vi "Update In World.vi"(11 "Chmmr in":refnum<class "Chmmr.lvclass">) -> (3 "Chmmr out":refnum<class "Chmmr.lvclass">)   [LabVIEW 2015, in "Chmmr.lvclass"]
uses:
  Chmmr.lvclass
  Element/Element.lvclass/Element.ctl
  Motion/Motion.lvclass/Motion.ctl
  Chmmr.lvclass/Chmmr.ctl
  <vilib>/Utility/High Resolution Relative Seconds.vi
  Ship/Ship.lvclass
  Math/Math.lvlib
  Motion/Motion.lvclass
  Element/Element.lvclass
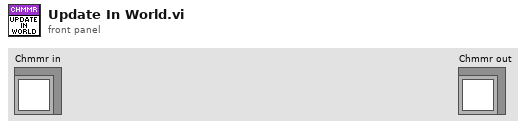
[diagram p1: front panel]
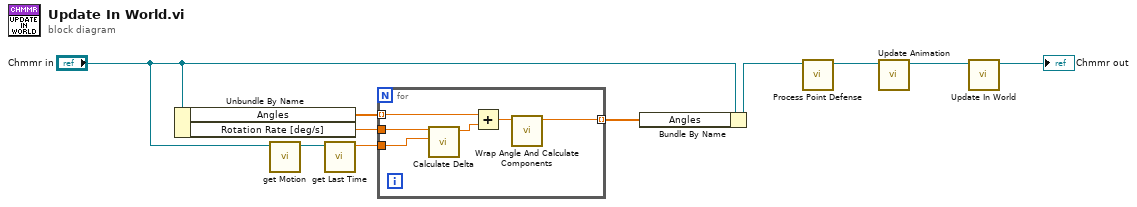
[diagram p0: block diagram]
diagram:
  n1 = Unbundle By Name("Chmmr in") -> ("Angles"=w10:sgl[], "Rotation Rate [deg/s]"=w8:sgl)
  n2 = call "get Motion.vi"("Movable in"="Chmmr in") -> ("Motion"=w7:refnum<class "Motion.lvclass">)  [unwired: 10 in]
  n3 = call "get Last Time.vi"("Motion in"=w7) -> ("Last Time"=w6:dbl)  [unwired: 10 in]
  n4 = for {
    tunnel: w10 -> [w14] mode=indexing
    tunnel: [w15] -> w9 mode=indexing
    tunnel: w6 -> [w16]
    tunnel: w8 -> [w13]
    n5 = call "Calculate Delta.vi"("Last Time"=w16, "Property"=w13) -> ("Delta"=w12:sgl)  [unwired: 9 in]
    n6 = Add(x=w14, y=w12) -> (x+y=w11:sgl)
    n7 = call "Wrap Angle And Calculate Components.vi"("Angle in [deg]"=w11) -> ("Angle out [deg]"=w15:sgl)  [unwired: 10 in]
  }
  n8 = Bundle By Name(cluster="Chmmr in", "Angles"=w9) -> (w2:refnum<class "Chmmr.lvclass">)
  n9 = call "Process Point Defense.vi"("Chmmr in"=w2) -> ("Chmmr out"=w1:refnum<class "Chmmr.lvclass">)  [unwired: 10 in]
  n10 = call "Update Animation.vi"("Chmmr in"=w1) -> ("Chmmr out"=w5:refnum<class "Chmmr.lvclass">)  [unwired: 10 in]
  n11 = call-parent "Update In World.vi"("Ship in"=w5) -> ("Ship out"=→"Chmmr out":refnum<class "Chmmr.lvclass">)  [unwired: 10 in]
